vi "Get Event Registration.vi"(8 "error in (no error)":errorcluster, 11 "Worker in":refnum<class "Worker.lvclass">) -> (0 "error out":errorcluster, 2 "Event Registration Refnum":refnum<event-registration>, 3 "Worker out":refnum<class "Worker.lvclass">)   [LabVIEW 2023, in "Worker.lvlib" / "Worker.lvclass"]
doc: "Create all User Events needed by the parent Worker UI."
uses:
  Worker.lvclass
  c:/dev/_r/4/eng/lv-core/lvpostprocessingd/lv_mc_x86_64/dist_i386/examples/Design Patterns/Actor Framework/Classes/Person/Person.lvclass
  Person/Person.lvclass/Person.ctl
  Worker.lvclass/Worker.ctl
  Person/Person.lvclass
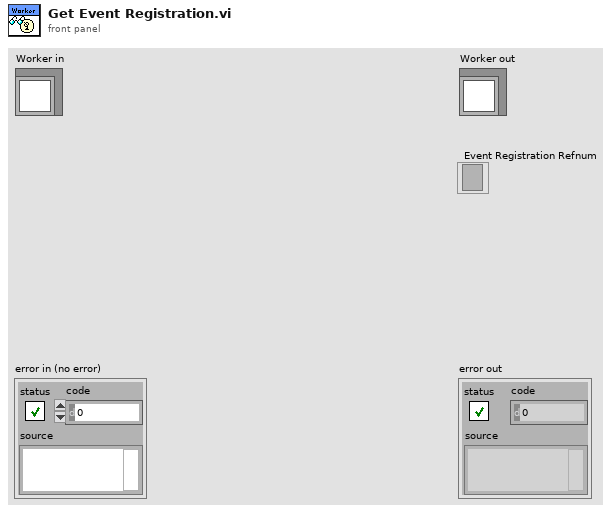
[diagram p1: front panel]
types:
  T1 = cluster{"Stop":refnum<user-event>, "Status":refnum<user-event>, "Count":refnum<user-event>}
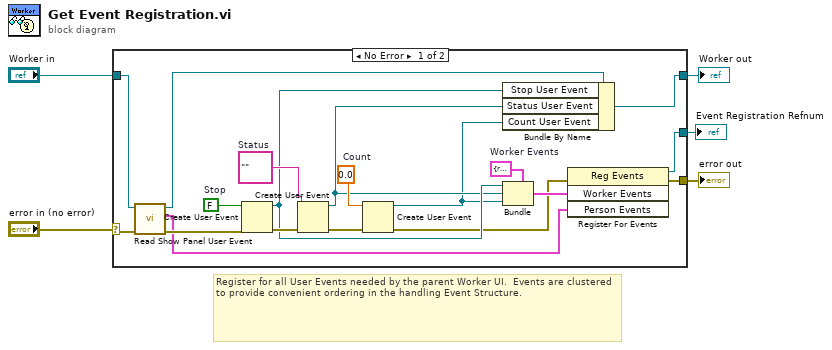
[diagram p0: block diagram]
diagram:
  # "Register for all User Events needed by the parent Worker UI.  Events are clustered to provide convenient ordering in the handling Event Structure."
  n1 = case shown="No Error" "error in (no error)" {
    selector: "error in (no error)" -> [w12 w26]
    tunnel: [w22 w26] -> w4
    tunnel: [w21 w25] -> w2
    tunnel: "Worker in" -> [w11 w25]
    tunnel: [w23 _] -> w1
    frame No Error {
      w7 = T1 {"Stop"=refnum, "Status"=refnum, "Count"=refnum}  # Worker Events
      w16 = 0.0  # Count
      w17 = ""  # Status
      w20 = FALSE  # Stop
      n2 = call "Read Show Panel User Event.vi"("error in (no error)"=w12, "Person in"=w11) -> ("error out"=w9:errorcluster, "Person Events"=w6:cluster{"Show Panel":refnum<user-event>}, "Person out"=w10:refnum<class "Worker.lvclass">)  [unwired: 7 in]
      n3 = Create User Event(user event datatype=w20, error in=w9) -> (user event=w15:refnum<user-event>, error out=w19:errorcluster)
      n4 = Create User Event(user event datatype=w17, error in=w19) -> (user event=w14:refnum<user-event>, error out=w18:errorcluster)
      n5 = Create User Event(user event datatype=w16, error in=w18) -> (user event=w13:refnum<user-event>, error out=w8:errorcluster)
      n6 = Bundle By Name(cluster=w10, "Stop User Event"=w15, "Status User Event"=w14, "Count User Event"=w13) -> (w21:refnum<class "Worker.lvclass">)
      n7 = Bundle(cluster=w7, "Stop"=w15, "Status"=w14, "Count"=w13) -> (w24:T1)
      n8 = register-events(error in=w8, w24, w6) -> (reference out=w23:refnum<event-registration>, error out=w22:errorcluster)  [unwired: 1 in]
    }
    frame Error {
    }
  }
  "error out" <- w4
  "Worker out" <- w2
  "Event Registration Refnum" <- w1
